vi "Write Test Timing.vi"(6 "Vacuum?":bool, 8 "error in (no error)":errorcluster, 11 "Test Configuration":T1) -> (0 "error out":errorcluster)   [LabVIEW 2015, in "UI Handler.lvclass"]
uses:
  UI Handler.lvclass
  Tests/Controls/Test Information.ctl
  Tests/Controls/Vacuum Test.ctl
  Tests/Controls/Test Timing.ctl
  Tests/Controls/Vaccum Thresholds.ctl
  Tests/Controls/Helium Test.ctl
  Tests/Controls/Helium Thresholds.ctl
  Tests/Controls/Startup Thresholds.ctl
  UI Handler.lvclass/UI Handler.ctl
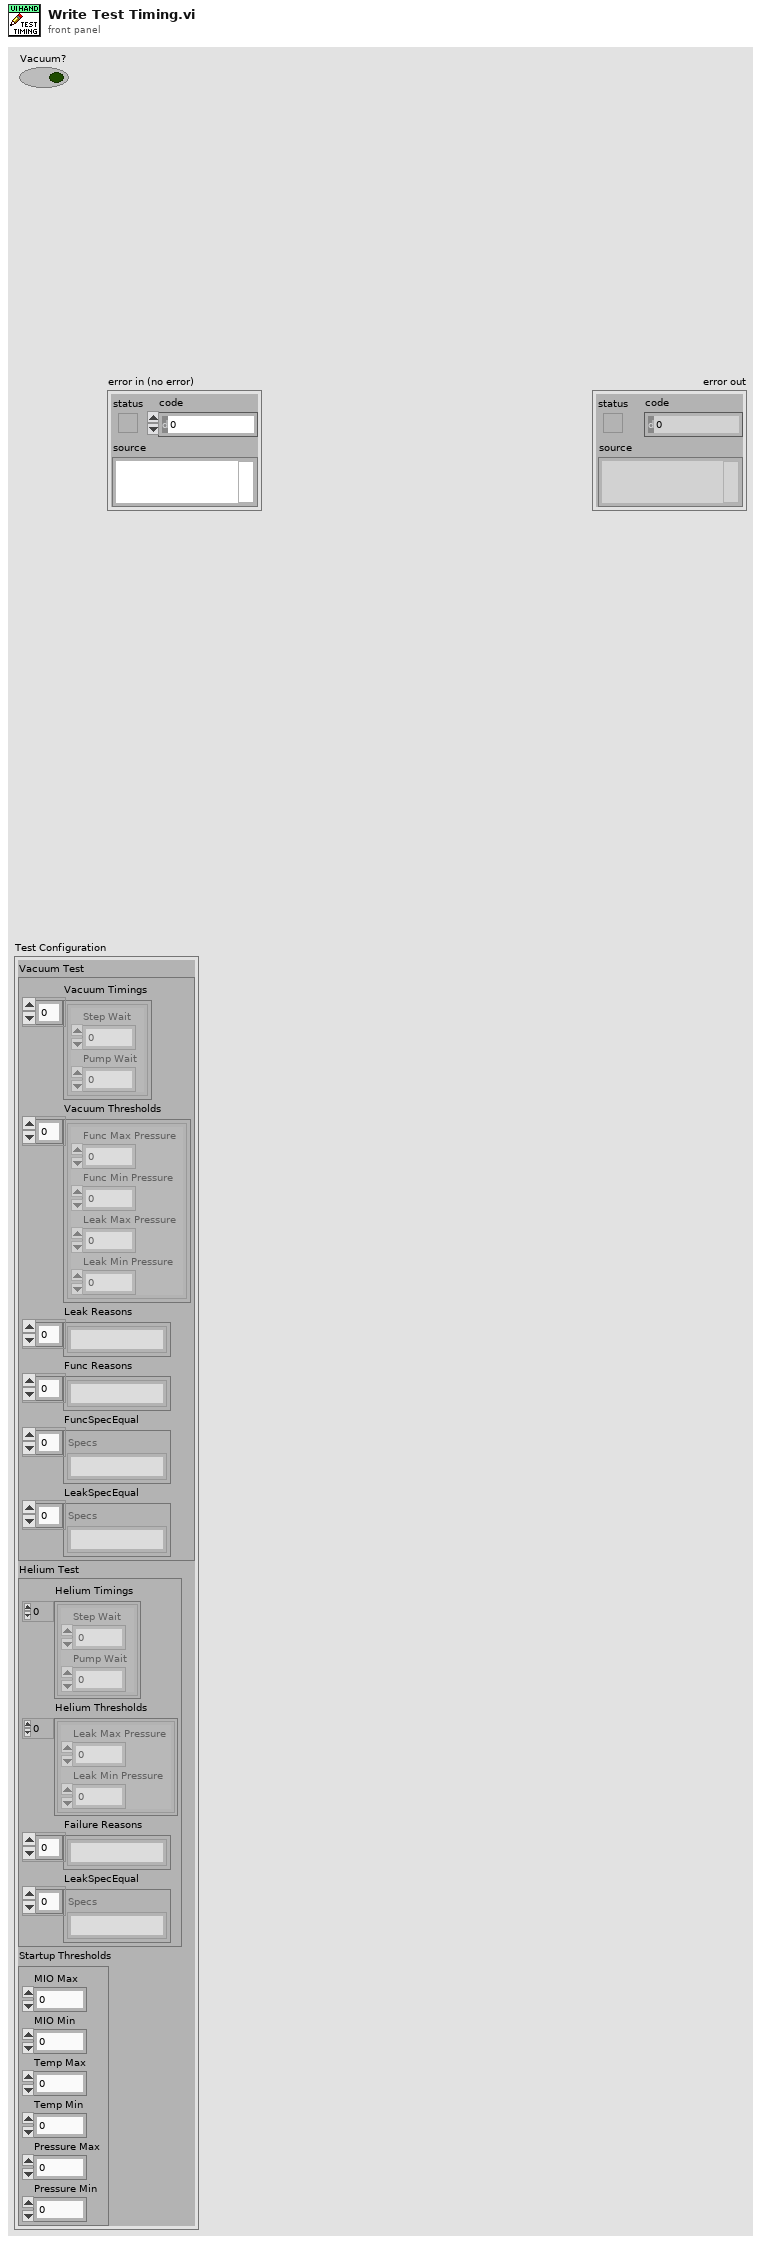
[diagram p1: front panel]
types:
  T1 = typedef "Test Information.ctl" = cluster{"Vacuum Test":T2, "Helium Test":T5, "Startup Thresholds":T7}
  T2 = typedef "Vacuum Test.ctl" = cluster{"Vacuum Timings":T3[], "Vacuum Thresholds":T4[], "Leak Reasons":string[], "Func Reasons":string[], "FuncSpecEqual":string[], "LeakSpecEqual":string[]}
  T3 = typedef "Test Timing.ctl" = cluster{"Step Wait":dbl, "Pump Wait":dbl}
  T4 = typedef "Vaccum Thresholds.ctl" = cluster{"Func Max Pressure":dbl, "Func Min Pressure":dbl, "Leak Max Pressure":dbl, "Leak Min Pressure":dbl}
  T5 = typedef "Helium Test.ctl" = cluster{"Helium Timings":T3[], "Helium Thresholds":T6[], "Failure Reasons":string[], "LeakSpecEqual":string[]}
  T6 = typedef "Helium Thresholds.ctl" = cluster{"Leak Max Pressure":dbl, "Leak Min Pressure":dbl}
  T7 = typedef "Startup Thresholds.ctl" = cluster{"MIO Max":dbl, "MIO Min":dbl, "Temp Max":dbl, "Temp Min":dbl, "Pressure Max":dbl, "Pressure Min":dbl}
  T8 = typedef "UI Handler.lvclass/Session Handle.ctl" = refnum<data-value>
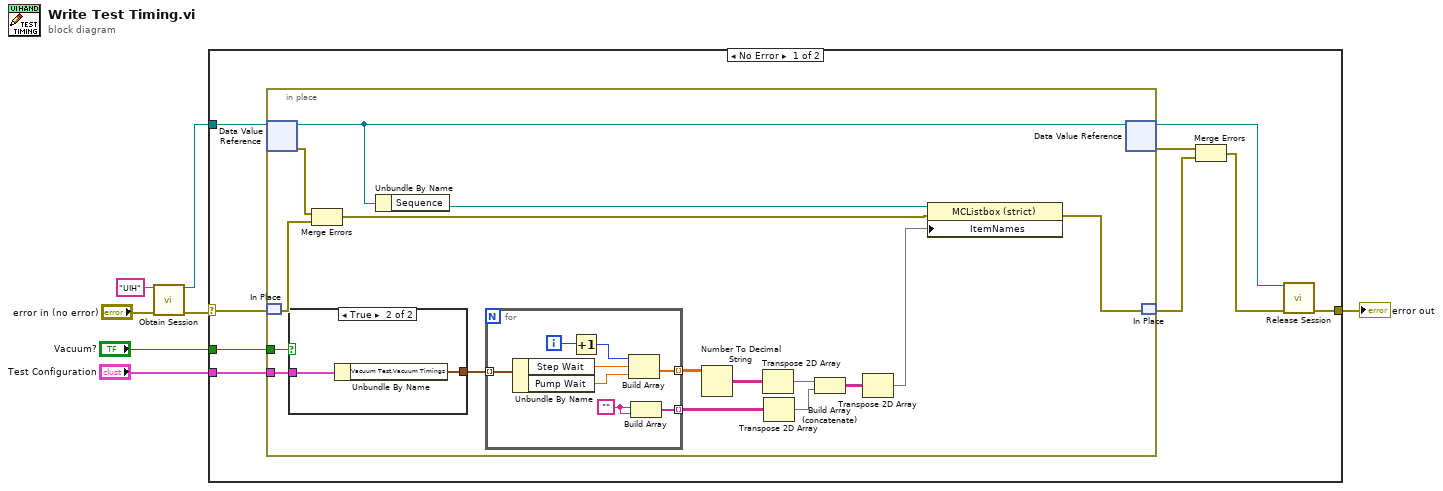
[diagram p0: block diagram]
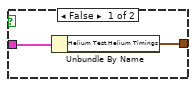
[diagram p2: hidden frame]
diagram:
  n1 = call "Obtain Session.vi"("Session  Name ()"="UIH", "error in (no error)"="error in (no error)") -> ("Session Handle"=w3:T8, "error out"=w4:errorcluster)  [unwired: 12 in]
  n2 = case shown="No Error" w4 {
    selector: w4 -> [w13 w45]
    tunnel: w3 -> [w16 _]
    tunnel: [w11 w45] -> w6
    tunnel: "Test Configuration" -> [w9 _]
    tunnel: "Vacuum?" -> [w8 _]
    frame No Error {
      n3 = in-place {
        in-place-border: w9 -> [w27]
        in-place-border: w8 -> [w28]
        n4 = in-place-dvr #1(w16) -> (w32:refnum<class "UI Handler.lvclass">, w31:errorcluster)
        n5 = in-place-match #2(w13) -> (w30:errorcluster)
        n6 = case shown="True" w28 {
          tunnel: w27 -> [w42 w44]
          tunnel: [w41 w43] -> w20
          frame False {
            n7 = Unbundle By Name(w42) -> ("Helium Test.Helium Timings"=w41:T3[])
          }
          frame True {
            n8 = Unbundle By Name(w44) -> ("Vacuum Test.Vacuum Timings"=w43:T3[])
          }
        }
        n9 = Merge Errors(w31, w30) -> (w18:errorcluster)
        n10 = Unbundle By Name(w32) -> ("Sequence"=w19:refnum<vi>)
        n11 = for {
          tunnel: w20 -> [w40] mode=indexing
          tunnel: [w37] -> w26 mode=indexing
          tunnel: [w33] -> w24 mode=indexing
          i -> [w36]
          w34 = ""
          n12 = Unbundle By Name(w40) -> ("Step Wait"=w39:dbl, "Pump Wait"=w38:dbl)
          n13 = Increment(x=w36) -> (x+1=w35:i32)
          n14 = Build Array(w35, w39, w38) -> (w37:dbl[])
          n15 = Build Array(w34, w34) -> (w33:string[])
        }
        n16 = Number To Decimal String(number=w26) -> (decimal integer string=w25:string[][])  [unwired: 1 in]
        n17 = Transpose 2D Array(2D array=w25) -> (transposed array=w23:string[][])
        n18 = Transpose 2D Array(2D array=w24) -> (transposed array=w22:string[][])
        n19 = Build Array (concatenate)(w23, w22) -> (w21:string[][])
        n20 = Transpose 2D Array(2D array=w21) -> (transposed array=w17:string[][])
        n21 = property on="Property Node" class="MCListbox (strict)"(reference=w19, error in=w18, "ItemNames"=w17) -> (error out=w29:errorcluster)  [unwired: 1 out]
        n22 = in-place-dvr #1(w32) -> (w10:T8, w14:errorcluster)
        n23 = in-place-match #2(w29) -> (w15:errorcluster)
      }
      n24 = Merge Errors(w14, w15) -> (w12:errorcluster)
      n25 = call "Release Session.vi"("Session Handle"=w10, "error in (no error)"=w12) -> ("error out"=w11:errorcluster)  [unwired: 13 in]
    }
    frame Error {
    }
  }
  "error out" <- w6
